vi "n x n Kernel Convolution (SGL).vi"(4 "Average":bool caption="Average (F)", 5 "Convolution Algorithm (direct)":enum32{"direct", "frequency domain"}(ring), 6 "Threshold Low":sgl=-inf, 7 "Threshold High":sgl=inf, 8 "Error In":errorcluster, 9 "Kernel Size":i32=1, 10 "Kernel Type":T1, 11 "Array in":sgl[][](array[numeric])) -> (0 "Error Out":errorcluster, 1 "Valid?":bool[][](array[boolean]), 3 "Array out":sgl[][](array[numeric]))   [LabVIEW 2021, in "Arrays.lvlib"]
uses:
  Arrays.lvlib
  Kernel Type.ctl
  <vilib>/Utility/error.llb/DialogType.ctl
  d0ebc029-cbaa-4c82-a58c-923c59c440da.vi
  b80d5e79-a0c8-46e2-aba9-3d60e0093a16.vi
  <vilib>/Analysis/2dsp.llb/2D Convolution (DBL).vi
  Time/Time.lvlib
  <vilib>/Analysis/NI_AALPro.lvlib
panel:
  out "elapsed (relative) seconds":dbl
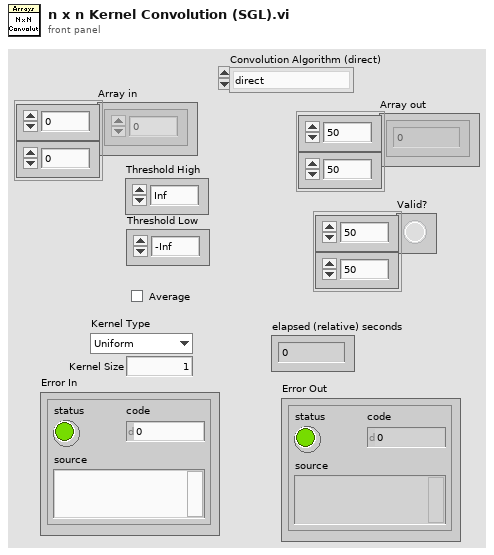
[diagram p1: front panel]
types:
  T1 = typedef "Arrays.lvlib/Kernel Type.ctl" = enum16{"Uniform", "Bilinear", "Gaussian"}
  T2 = typedef "DialogType.ctl" = u16
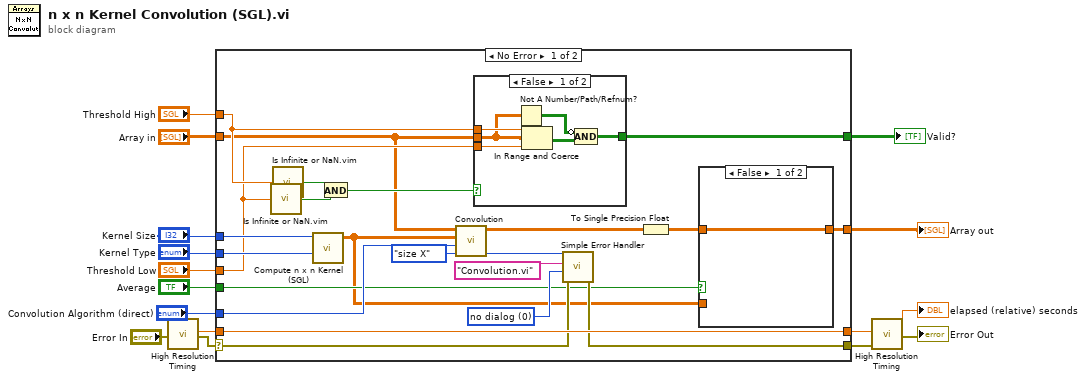
[diagram p0: block diagram]
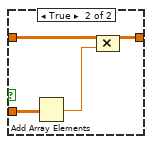
[diagram p2: hidden frame]
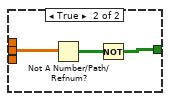
[diagram p3: hidden frame]
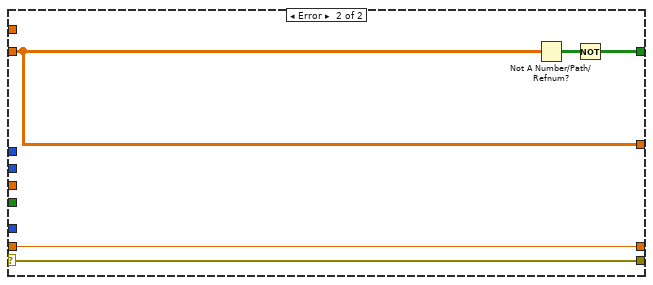
[diagram p4: hidden frame]
diagram:
  n1 = call "High Resolution Timing.vi"("Error In"="Error In") -> ("elapsed (relative) seconds"=w5:dbl, "Error Out"=w6:errorcluster)  [unwired: 16 in, 1 out]
  n2 = case shown="No Error" w6 {
    selector: w6 -> [w23 w53]
    tunnel: "Array in" -> [w29 w56]
    tunnel: "Kernel Size" -> [w38 _]
    tunnel: [w18 w56] -> w15
    tunnel: "Threshold Low" -> [w32 _]
    tunnel: "Threshold High" -> [w33 _]
    tunnel: [w30 w55] -> w14
    tunnel: [w36 w54] -> w3
    tunnel: "Kernel Type" -> [w37 _]
    tunnel: "Average" -> [w21 _]
    tunnel: w5 -> [w36 w54]
    tunnel: "Convolution Algorithm (direct)" -> [w28 _]
    tunnel: [w22 w53] -> w1
    frame No Error {
      w24 = T2 0 items=["no dialog", "OK message", "continue or stop message", "OK message + warnings", "continue/stop + warnings"] ("type of dialog (OK msg:1)")
      n3 = call "Is Infinite or NaN.vim"("Number"=w32) -> ("Is NaN or Inf?"=w35:bool)  [unwired: 8 in]
      n4 = call "Is Infinite or NaN.vim"("Number"=w33) -> ("Is NaN or Inf?"=w34:bool)  [unwired: 8 in]
      n5 = call "Compute n x n Kernel (SGL).vi"("Kernel Type"=w37, "Kernel Size"=w38) -> ("Kernel"=w19:sgl[][])  [unwired: 9 in]
      n6 = And(x=w34, y=w35) -> (x .and. y?=w31:bool)
      n7 = call-poly <vilib>:"Convolution.vi"("output size"=enum32{"full", "size X", "compact"}."size X", "algorithm"=w28, "Y"=w19, "X"=w29) -> ("error"=w26:i32, "X * Y"=w20:dbl[][])  [unwired: 6 in]
      n8 = case shown="False" w31 {
        tunnel: w33 -> [w47 _]
        tunnel: w32 -> [w46 _]
        tunnel: w29 -> [w45 w52]
        tunnel: [w44 w50] -> w30
        frame False {
          n9 = Not A Number/Path/Refnum?(number/path/refnum=w45) -> (NaN/Path/Refnum?=w49:bool[][])
          n10 = In Range and Coerce(upper limit=w47, x=w45, lower limit=w46) -> (In Range?=w48:bool[][])  [unwired: 1 out]
          n11 = Compound Arithmetic op=AND(invert w49, w48) -> (w44:bool[][])
        }
        frame True {
          n12 = Not A Number/Path/Refnum?(number/path/refnum=w52) -> (NaN/Path/Refnum?=w51:bool[][])
          n13 = Not(x=w51) -> (.not. x?=w50:bool[][])
        }
      }
      n14 = call <vilib>:"Simple Error Handler.vi"("error code (no error:0)"=w26, "error source (\" \")"="Convolution.vi" ("error source (\" \")"), "type of dialog (OK msg:1)"=w24, "error in (no error)"=w23) -> ("error out"=w22:errorcluster)  [unwired: 1 in, 4 out]
      n15 = To Single Precision Float(number=w20) -> (single precision float=w17:sgl[][])
      n16 = case shown="False" w21 {
        tunnel: w17 -> [w39 w42]
        tunnel: w19 -> [_ w43]
        tunnel: [w39 w40] -> w18
        frame False {
        }
        frame True {
          n17 = Add Array Elements(numeric array=w43) -> (sum=w41:sgl)
          n18 = Compound Arithmetic op=MULTIPLY(w42, w41) -> (w40:sgl[][])
        }
      }
    }
    frame Error {
      n19 = Not A Number/Path/Refnum?(number/path/refnum=w56) -> (NaN/Path/Refnum?=w57:bool[][])
      n20 = Not(x=w57) -> (.not. x?=w55:bool[][])
    }
  }
  "Array out" <- w15
  "Valid?" <- w14
  n21 = call "High Resolution Timing.vi"("relative seconds (NaN)"=w3, "Error In"=w1) -> ("elapsed (relative) seconds"=→"elapsed (relative) seconds":dbl, "Error Out"=→"Error Out":errorcluster)  [unwired: 15 in, 1 out]
